vi "Initialize.vi"(7 "error in":errorcluster caption="错误输入（无错误）", 10 "PanelDataNode in":refnum<class "PanelDataNode.lvclass"> caption="LinkNode in") -> (0 "error out":errorcluster caption="错误输出", 2 "SelfNode*":refnum<data-value>)   [LabVIEW 2013, in "PanelDataNode.lvclass"]
uses:
  PanelDataNode.lvclass
  PanelLinkNode/PanelLinkNode.lvclass
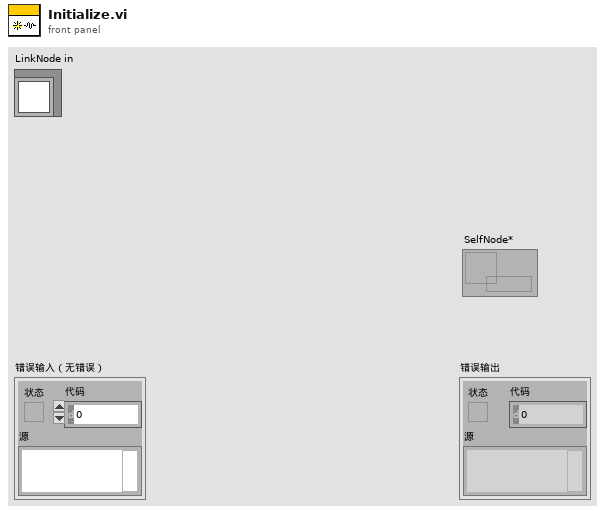
[diagram p1: front panel]
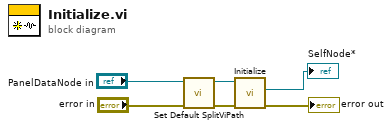
[diagram p0: block diagram]
diagram:
  n1 = call-dynamic "Set Default SplitViPath.vi"("error in (no error)"="error in", "PanelDataNode 输入"="PanelDataNode in") -> ("error out"=w2:errorcluster, "PanelDataNode 输出"=w3:refnum<class "PanelDataNode.lvclass">)  [unwired: 8 in]
  n2 = call-parent "Initialize.vi"("error in (no error)"=w2, "PanelLinkNode 输入"=w3) -> ("error out"=→"error out":errorcluster, "SelfNode*"=→"SelfNode*":refnum<data-value>)  [unwired: 7 in]
